vi "Config File View-DS.vi"(10 "File View":bool, 11 "Path":path) -> (0 "refnum out":refnum<file>, 1 "FCS Version Name":string, 2 "Cancel Button Ind":bool, 4 "error out":errorcluster)   [LabVIEW 2020]
panel:
  in  "Cancel Button":bool
  in  "OK Button":bool
  in  "Text Ring":u16(ring) items=["Struct2 ", "Structure1 ", "Structure2 "]
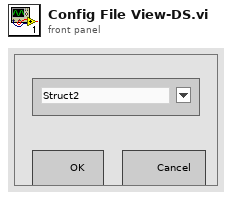
[diagram p1: front panel]
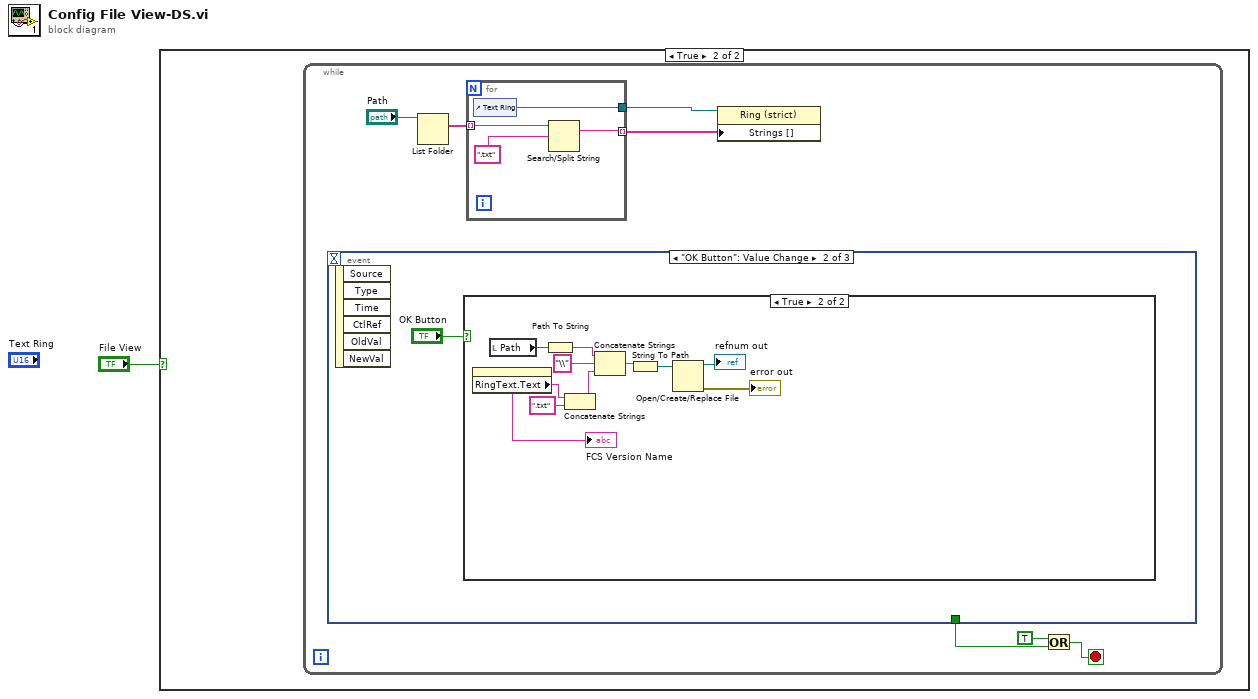
[diagram p0: block diagram]
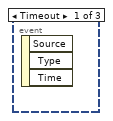
[diagram p3: hidden frame]
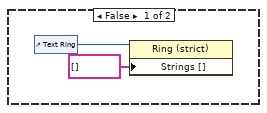
[diagram p4: hidden frame]
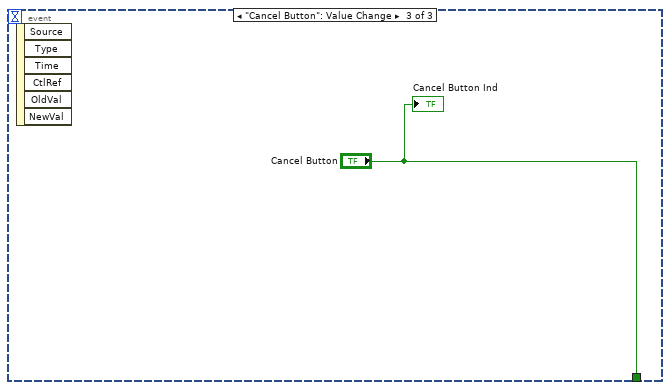
[diagram p5: hidden frame]
diagram:
  n1 = case shown="True" "File View" {
    frame False {
    }
    frame True {
      n2 = while {
        stop <- w7 stop-if-true
        n3 = event shown="[1] \"OK Button\": Value Change" {
          selector: _ -> [_ _ _]
          dyn-events: _ -> [_ _ _]
          timeout: _ -> [_ _ _]
          tunnel: [_ _ "Cancel Button"] -> w4
          event Timeout {
            n4 = event-data() -> ()  [unwired: 1 in, 3 out]
          }
          event "OK Button": Value Change {
            n5 = event-data() -> ()  [unwired: 1 in, 6 out]
            n6 = case shown="True" "OK Button" {
              frame False {
                n7 = control-ref of="Text Ring"() -> (w14:refnum<vi>)
                n8 = property on="Property Node" class="Ring (strict)"(reference=w14, "Strings []"=string[] []) -> ()  [unwired: 1 in, 2 out]
              }
              frame True {
                n9 = property on="Text Ring" class="Ring (strict)"() -> ("RingText.Text"=w18:string)  [unwired: 2 in, 2 out]
                "FCS Version Name" <- w18
                n10 = local read "Path"() -> (w25:path)
                n11 = Path To String(path=w25) -> (string=w24:string)
                n12 = Concatenate Strings(w18, ".txt" ("string")) -> (w16:string)
                n13 = Concatenate Strings(w24, "\\" ("string"), w16) -> (w22:string)
                n14 = String To Path(string=w22) -> (path=w21:path)
                n15 = Open/Create/Replace File(file path (use dialog)=w21) -> (refnum out=→"refnum out":refnum<file>, error out=→"error out":errorcluster)  [unwired: 5 in, 1 out]
              }
            }
          }
          event "Cancel Button": Value Change {
            n16 = event-data() -> ()  [unwired: 1 in, 6 out]
            "Cancel Button Ind" <- "Cancel Button"
          }
        }
        n17 = List Folder(path="Path") -> (filenames=w6:string[])  [unwired: 3 in, 3 out]
        n18 = for {
          tunnel: w6 -> [w12] mode=indexing
          tunnel: [w10] -> w3
          tunnel: [w9] -> w2 mode=indexing
          n19 = control-ref of="Text Ring"() -> (w10:refnum<vi>)
          n20 = Search/Split String(string=w12, search string/char (-)=".txt") -> (substring before match=w9:string)  [unwired: 1 in, 2 out]
        }
        n21 = property on="Property Node" class="Ring (strict)"(reference=w3, "Strings []"=w2) -> ()  [unwired: 1 in, 2 out]
        n22 = Or(x=TRUE, y=w4) -> (x .or. y?=w7:bool)
      }
    }
  }
